vi "Manage Camera.vi"(9 "Choose Camera":u16, 10 "Camera IDs":string[](array[string]), 11 "Image in":T1) -> (3 "Image out":T1)   [LabVIEW 2025]
uses:
  <vilib>/vision/Image Controls.llb/IMAQ Image.ctl
  488ee405-1aa7-4078-ab1d-4b9aa6deceb3.vi
  <vilib>/vision/driver/NI_Vision_Acquisition_Software.lvlib
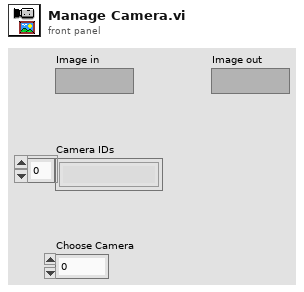
[diagram p1: front panel]
types:
  T1 = typedef "IMAQ Image.ctl" = refnum<image>
  T2 = typedef "IMAQdx.ctl" = refnum<k21>
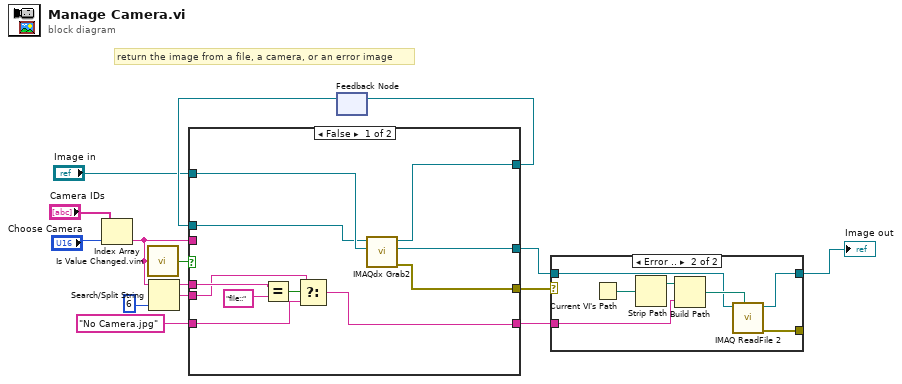
[diagram p0: block diagram]
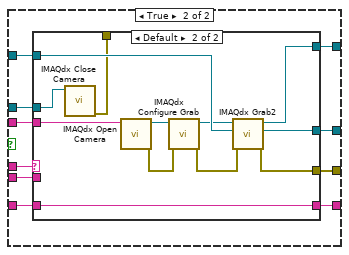
[diagram p3: hidden frame]
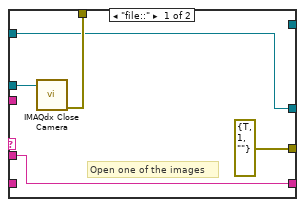
[diagram p4: hidden frame]
diagram:
  # "return the image from a file, a camera, or an error image"
  n1 = Index Array(array="Camera IDs", index="Choose Camera") -> (element=w4:string)
  n2 = call "Is Value Changed.vim"("value"=w4) -> ("changed or first call?"=w13:bool)
  n3 = Search/Split String(string=w4, offset (0)=6 ("length (rest)")) -> (substring before match=w2:string, match + rest of string=w1:string)  [unwired: 1 in, 1 out]
  n4 = feedback #1() -> (w15:T2)  [unwired: 1 in]
  n5 = case shown="False" w13 {
    tunnel: [w25 w36] -> w14
    tunnel: w15 -> [w24 w33]
    tunnel: w4 -> [_ w34]
    tunnel: [w22 w35] -> w8
    tunnel: "Image in" -> [w26 w32]
    tunnel: [w23 w31] -> w9
    tunnel: "No Camera.jpg" -> [w16 w29]
    tunnel: [w17 w30] -> w5
    tunnel: w2 -> [w21 w28]
    tunnel: w1 -> [w18 w27]
    frame False {
      n6 = Equal?(x=w21, y="file::") -> (x = y?=w19:bool)
      n7 = Select(t=w18, s=w19, f=w16) -> (s? t:f=w17:string)
      n8 = call <vilib>:"IMAQdx Grab2.vi"("Image In"=w26, "Session In"=w24) -> ("error out"=w22:errorcluster, "Image Out"=w23:T1, "Session Out"=w25:T2)  [unwired: 6 in, 1 out]
    }
    frame True {
      n9 = case shown="Default" w28 {
        tunnel: [_ w47] -> w36
        tunnel: w34 -> [_ w51]
        tunnel: [errorcluster {"status"=TRUE, "code"=1, "source"=""} ("error out") w45] -> w35
        tunnel: w27 -> [w38 _]
        tunnel: w33 -> [w41 w50]
        tunnel: w32 -> [w39 w49]
        tunnel: [w39 w44] -> w31
        tunnel: [w40 w43] -> _
        tunnel: [w38 w42] -> w30
        tunnel: w29 -> [_ w42]
        frame "file::" {
          # "Open one of the images"
          n10 = call <vilib>:"IMAQdx Close Camera.vi"("Session In"=w41) -> ("error out"=w40:errorcluster)  [unwired: 10 in]
        }
        frame Default {
          n11 = call <vilib>:"IMAQdx Close Camera.vi"("Session In"=w50) -> ("error out"=w43:errorcluster)  [unwired: 10 in]
          n12 = call <vilib>:"IMAQdx Open Camera.vi"("Session In"=w51) -> ("error out"=w52:errorcluster, "Session Out"=w53:T2)  [unwired: 9 in]
          n13 = call <vilib>:"IMAQdx Configure Grab.vi"("error in"=w52, "Session In"=w53) -> ("error out"=w46:errorcluster, "Session Out"=w48:T2)  [unwired: 8 in]
          n14 = call <vilib>:"IMAQdx Grab2.vi"("error in"=w46, "Image In"=w49, "Session In"=w48) -> ("error out"=w45:errorcluster, "Image Out"=w44:T1, "Session Out"=w47:T2)  [unwired: 5 in, 1 out]
        }
      }
    }
  }
  n15 = feedback-in #1(w14) -> ()
  n16 = case shown="Error .." w8 {
    tunnel: w9 -> [w54 w58]
    tunnel: [w54 w57] -> w7
    tunnel: [_ w56] -> _
    tunnel: w5 -> [_ w55]
    frame No Error {
    }
    frame Error {
      n17 = Current VI's Path() -> (path=w60:path)
      n18 = Strip Path(path=w60) -> (stripped path=w61:path)  [unwired: 1 out]
      n19 = Build Path(base path=w61, name or relative path=w55) -> (appended path=w59:path)
      n20 = call "IMAQ ReadFile 2"("File Path"=w59, "Image"=w58) -> ("error out"=w56:errorcluster, "Image Out"=w57:T1)  [unwired: 5 in, 3 out]
    }
  }
  "Image out" <- w7
